vi "Run.vi"(8 "error in (no error)":errorcluster, 11 "GSstatus in":refnum<class "GSstatus.lvclass">) -> (0 "error out":errorcluster, 3 "GSstatus out":refnum<class "GSstatus.lvclass">)   [LabVIEW 2018, in "GSstatus.lvclass"]
uses:
  GSstatus.lvclass
  GSstatus.lvclass/GSstatus.ctl
  Device/Device.lvclass
  StateMachine/State Machine.lvclass
panel:
  in  "GS STATUS cluster":T1
  out "GS erro":errorcluster
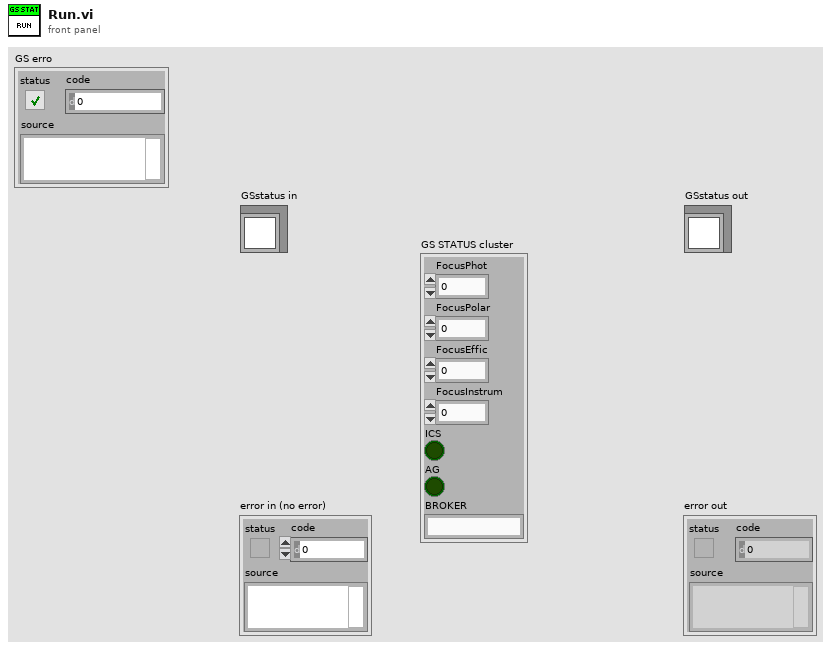
[diagram p1: front panel]
types:
  T1 = cluster{"FocusPhot":dbl, "FocusPolar":dbl, "FocusEffic":dbl, "FocusInstrum":dbl, "ICS":bool, "AG":bool, "BROKER":string}
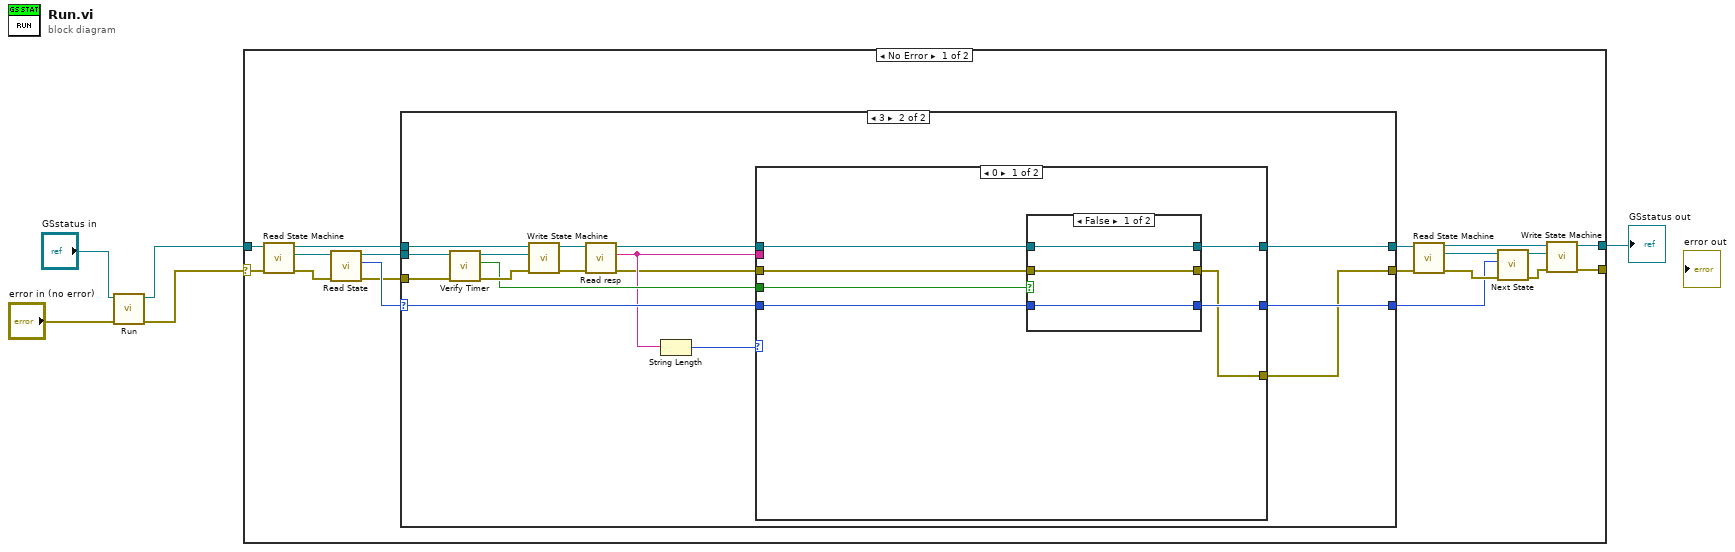
[diagram p0: block diagram]
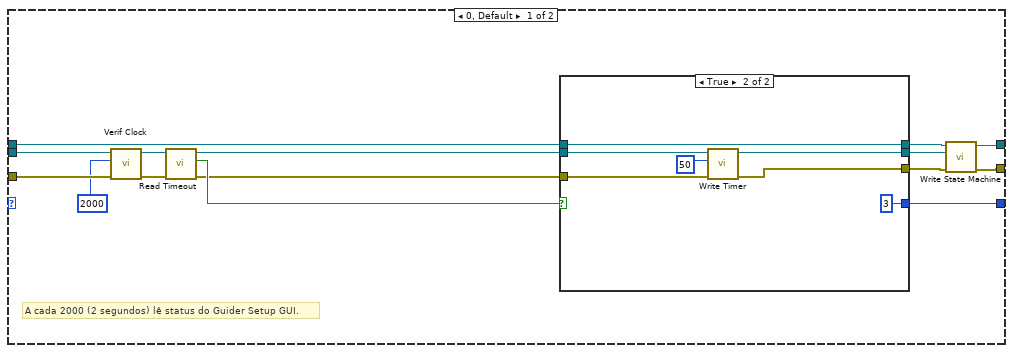
[diagram p2: hidden frame]
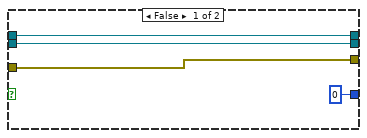
[diagram p3: hidden frame]
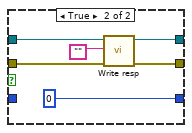
[diagram p4: hidden frame]
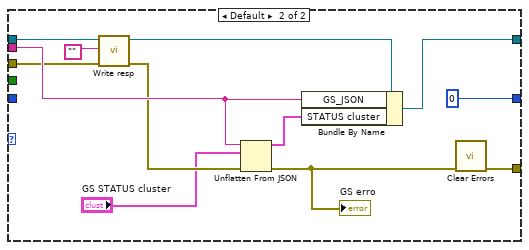
[diagram p5: hidden frame]
diagram:
  n1 = call-parent "Run.vi"("error in (no error)"="error in (no error)", "Device in"="GSstatus in") -> ("error out"=w2:errorcluster, "Device out"=w3:refnum<class "GSstatus.lvclass">)  [unwired: 8 in]
  n2 = case shown="No Error" w2 {
    selector: w2 -> [w22 w95]
    tunnel: [w14 w95] -> _
    tunnel: w3 -> [w23 w94]
    tunnel: [w13 w94] -> w1
    frame No Error {
      n3 = call-dynamic "Read State Machine.vi"("error in (no error)"=w22, "Device in"=w23) -> ("error out"=w20:errorcluster, "State Machine.lvclass"=w21:refnum<class "State Machine.lvclass">, "Device out"=w11:refnum<class "GSstatus.lvclass">)  [unwired: 7 in]
      n4 = call-dynamic "Read State.vi"("error in (no error)"=w20, "State Machine in"=w21) -> ("error out"=w10:errorcluster, "State"=w12:i32, "State Machine out"=w6:refnum<class "State Machine.lvclass">)  [unwired: 7 in]
      n5 = case shown="3" w12 {
        selector: w12 -> [_ w55]
        tunnel: w11 -> [w31 w60]
        tunnel: w10 -> [w37 w58]
        tunnel: [w25 w50] -> w9
        tunnel: [w24 w64] -> w8
        tunnel: [w32 w63] -> w7
        tunnel: w6 -> [w36 w62]
        frame 0, Default {
          # "A cada 2000 (2 segundos) lê status do Guider Setup GUI."
          n6 = call-dynamic "Verif Clock.vi"("error in (no error)"=w37, "period (ms)"=u32 2000 ("period"), "State Machine in"=w36) -> ("error out"=w38:errorcluster, "State Machine out"=w35:refnum<class "State Machine.lvclass">)  [unwired: 6 in, 1 out]
          n7 = call-dynamic "Read Timeout.vi"("error in (no error)"=w38, "State Machine in"=w35) -> ("error out"=w27:errorcluster, "Timeout"=w33:bool, "State Machine out"=w28:refnum<class "State Machine.lvclass">)  [unwired: 7 in]
          n8 = case shown="True" w33 {
            tunnel: [0 ("State") 3 ("State")] -> w32
            tunnel: w31 -> [w40 w49]
            tunnel: w27 -> [w41 w45]
            tunnel: [w41 w44] -> w26
            tunnel: [w40 w49] -> w30
            tunnel: [w39 w48] -> w29
            tunnel: w28 -> [w39 w47]
            frame False {
            }
            frame True {
              n9 = call-dynamic "Write Timer.vi"("error in (no error)"=w45, "Timer"=u32 50, "State Machine in"=w47) -> ("error out"=w44:errorcluster, "State Machine out"=w48:refnum<class "State Machine.lvclass">)  [unwired: 7 in]
            }
          }
          n10 = call-dynamic "Write State Machine.vi"("error in (no error)"=w26, "State Machine.lvclass"=w29, "Device in"=w30) -> ("error out"=w25:errorcluster, "Device out"=w24:refnum<class "GSstatus.lvclass">)  [unwired: 7 in]
        }
        frame 3 {
          n11 = call "Verify Timer.vi"("error in (no error)"=w58, "State Machine in"=w62) -> ("error out"=w59:errorcluster, "timeout"=w54:bool, "State Machine out"=w61:refnum<class "State Machine.lvclass">)  [unwired: 7 in]
          n12 = call-dynamic "Write State Machine.vi"("error in (no error)"=w59, "State Machine.lvclass"=w61, "Device in"=w60) -> ("error out"=w56:errorcluster, "Device out"=w57:refnum<class "GSstatus.lvclass">)  [unwired: 7 in]
          n13 = call-dynamic "Read resp.vi"("error in (no error)"=w56, "Device in"=w57) -> ("error out"=w51:errorcluster, "resp"=w52:string, "Device out"=w65:refnum<class "GSstatus.lvclass">)  [unwired: 7 in]
          n14 = String Length(string=w52) -> (length=w53:i32)
          n15 = case shown="0" w53 {
            tunnel: w65 -> [w69 w93]
            tunnel: [w68 w86] -> w64
            tunnel: [w71 0 ("State")] -> w63
            tunnel: w55 -> [w72 _]
            tunnel: w54 -> [w70 _]
            tunnel: w52 -> [_ w90]
            tunnel: w51 -> [w67 w88]
            tunnel: [w66 w84] -> w50
            frame 0 {
              n16 = case shown="False" w70 {
                tunnel: w72 -> [w75 _]
                tunnel: [w75 0 ("State")] -> w71
                tunnel: [w73 w78] -> w68
                tunnel: w69 -> [w73 w79]
                tunnel: w67 -> [w74 w77]
                tunnel: [w74 w76] -> w66
                frame False {
                }
                frame True {
                  n17 = call-dynamic "Write resp.vi"("error in (no error)"=w77, "resp"="", "Device in"=w79) -> ("error out"=w76:errorcluster, "Device out"=w78:refnum<class "GSstatus.lvclass">)  [unwired: 7 in]
                }
              }
            }
            frame Default {
              n18 = call-dynamic "Write resp.vi"("error in (no error)"=w88, "resp"="", "Device in"=w93) -> ("error out"=w87:errorcluster, "Device out"=w92:refnum<class "GSstatus.lvclass">)  [unwired: 7 in]
              n19 = Unflatten From JSON(JSON string=w90, type and defaults="GS STATUS cluster", error in (no error)=w87) -> (value=w82:T1, error out=w85:errorcluster)  [unwired: 4 in]
              "GS erro" <- w85
              n20 = Bundle By Name(cluster=w92, "GS_JSON"=w90, "STATUS cluster"=w82) -> (w86:refnum<class "GSstatus.lvclass">)
              n21 = call <vilib>:"Clear Errors.vi"("error in (no error)"=w85) -> ("error out"=w84:errorcluster)  [unwired: 5 in, 1 out]
            }
          }
        }
      }
      n22 = call-dynamic "Read State Machine.vi"("error in (no error)"=w9, "Device in"=w8) -> ("error out"=w16:errorcluster, "State Machine.lvclass"=w18:refnum<class "State Machine.lvclass">, "Device out"=w17:refnum<class "GSstatus.lvclass">)  [unwired: 7 in]
      n23 = call "Next State.vi"("error in (no error)"=w16, "New_State"=w7, "State Machine in"=w18) -> ("error out"=w15:errorcluster, "State Machine out"=w19:refnum<class "State Machine.lvclass">)  [unwired: 7 in]
      n24 = call-dynamic "Write State Machine.vi"("error in (no error)"=w15, "State Machine.lvclass"=w19, "Device in"=w17) -> ("error out"=w14:errorcluster, "Device out"=w13:refnum<class "GSstatus.lvclass">)  [unwired: 7 in]
    }
    frame Error {
    }
  }
  "GSstatus out" <- w1
